vi "Configure Analog Alarm Settings.vi"(0 "VISA resource name":refnum<visa-resource-name>, 1 "Unit Address (1)":u8=1 min=1 max=254, 2 "Alarm Number (1)":u16=1 min=1 max=4, 5 "Threshold (0)":u16 max=9999, 7 "Alarm Hysteresis (1)":u16=1 min=1 max=9999, 9 "Latching Mode (0: No Latch)":u16(ring) items=["No Latch", "Automatic Latching", "Manual Latching", "Event Latching"], 11 "error in (no error)":errorcluster, 12 "Enable Alarm Blocking (False: Disable)":bool, 13 "Enable Hysteresis (False: Disable)":bool=TRUE) -> (4 "VISA resource name out":refnum<visa-resource-name>, 15 "error out":errorcluster)   [LabVIEW 2010, in "Eurotherm 32xx Series.lvlib"]
doc: "This VI Configure parameters of selected analog alarm."
uses:
  <instrlib>/Eurotherm 32xx Series/Eurotherm 32xx Series.lvlib
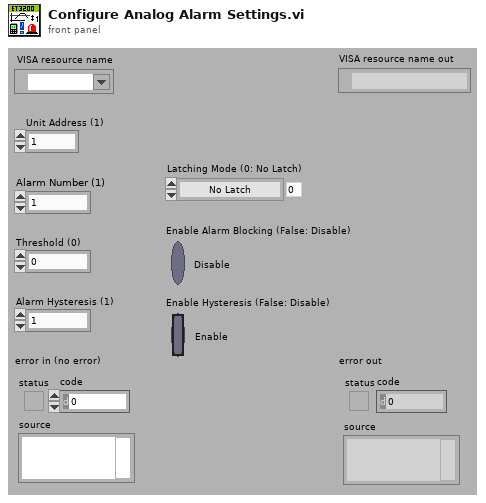
[diagram p1: front panel]
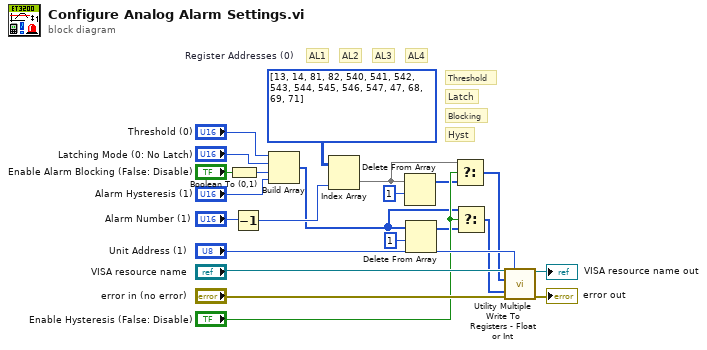
[diagram p0: block diagram]
diagram:
  w10 = u16[][] [[13, 14, 81, 82], [540, 541, 542, 543], [544, 545, 546, 547], [47, 68, 69, 71]]  # Register Addresses (0)
  # "Blocking"
  # "AL1"
  # "AL2"
  # "AL3"
  # "AL4"
  # "Latch"
  # "Hyst"
  # "Threshold"
  n1 = Boolean To (0,1)(Boolean="Enable Alarm Blocking (False: Disable)") -> (0, 1=w12:i16)
  n2 = Decrement(x="Alarm Number (1)") -> (x-1=w15:u16)
  n3 = Build Array("Threshold (0)", "Latching Mode (0: No Latch)", w12, "Alarm Hysteresis (1)") -> (w3:u16[])
  n4 = Index Array(array=w10, index (col)=w15) -> (element=w1:u16[])  [unwired: 1 in]
  n5 = Delete From Array(array=w1, length=1) -> (array with subset deleted=w2:u16[])  [unwired: 1 in, 1 out]
  n6 = Delete From Array(array=w3, length=1) -> (array with subset deleted=w4:u16[])  [unwired: 1 in, 1 out]
  n7 = Select(t=w1, s="Enable Hysteresis (False: Disable)", f=w2) -> (s? t:f=w7:u16[])
  n8 = Select(t=w3, s="Enable Hysteresis (False: Disable)", f=w4) -> (s? t:f=w6:u16[])
  n9 = call <instrlib>:"Utility Multiple Write To Registers - Float or Int.vi"("VISA resource name"="VISA resource name", "Unit Address (1)"="Unit Address (1)", "Registers Addresses (0)"=w7, "Data (0)"=w6, "error in (no error)"="error in (no error)") -> ("VISA resource name out"=→"VISA resource name out":refnum<visa-resource-name>, "error out"=→"error out":errorcluster)  [unwired: 9 in]
